vi "loopStop.vi"(8 "error in (no error)":errorcluster, 11 "Pixelfly in":refnum<class "PixelflySA.lvclass">) -> (0 "error out":errorcluster, 3 "Pixelfly out":refnum<class "PixelflySA.lvclass">)   [LabVIEW 2009, in "PixelflySA.lvclass"]
uses:
  PixelflySA.lvclass
  PixelflySA.lvclass/PixelflySA.ctl
  Channels.lvlib
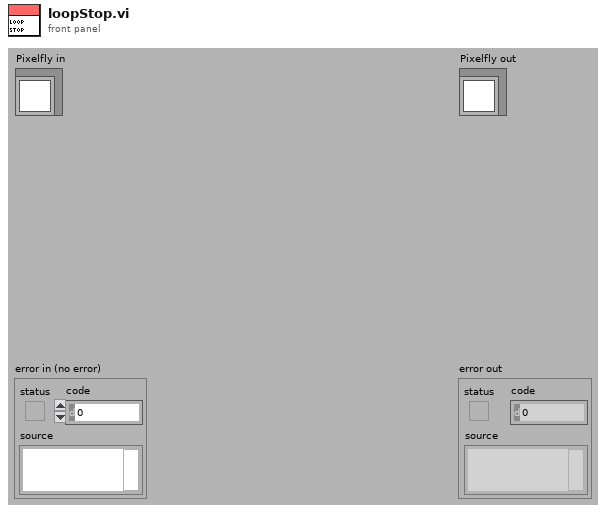
[diagram p1: front panel]
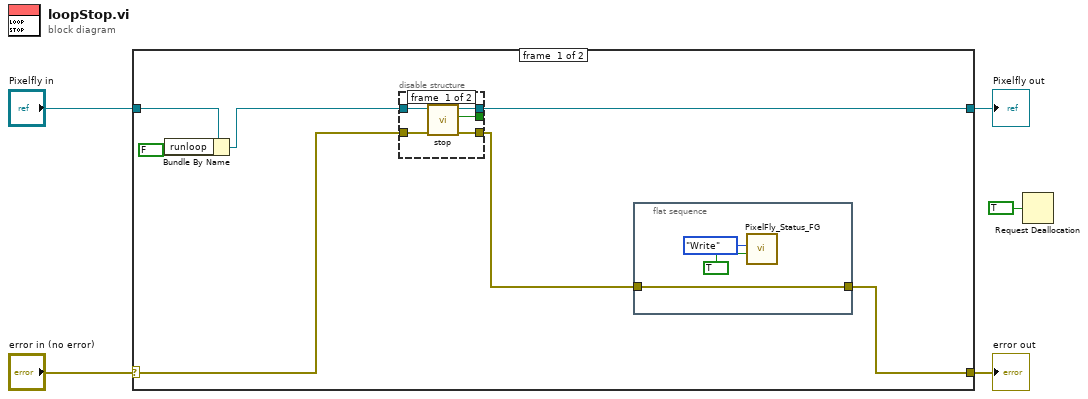
[diagram p0: block diagram]
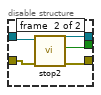
[diagram p2: hidden frame]
diagram:
  n1 = case shown="No Error" "error in (no error)" {
    selector: "error in (no error)" -> [w12 w27]
    tunnel: [w6 w27] -> w4
    tunnel: [w11 w26] -> w2
    tunnel: "Pixelfly in" -> [w9 w26]
    frame #0 {
      n2 = Bundle By Name(cluster=w9, "runloop"=FALSE) -> (w8:refnum<class "PixelflySA.lvclass">)
      n3 = disable-structure shown="Enabled" {
        disable-tunnel: w12 -> [w20 w23]
        disable-tunnel: [w19 w21] -> w7
        disable-tunnel: [w18 w22] -> _
        disable-tunnel: [w17 w25] -> w11
        disable-tunnel: w8 -> [w16 w24]
        frame #0 {
          n4 = call-dynamic "stop.vi"("error in (no error)"=w20, "Pixelfly in"=w16) -> ("error out"=w19:errorcluster, "stopped?"=w18:bool, "Pixelfly out"=w17:refnum<class "PixelflySA.lvclass">)  [unwired: 6 in, 1 out]
        }
        frame #1 {
          n5 = call-dynamic "stop2.vi"("error in (no error)"=w23, "Pixelfly in"=w24) -> ("error out"=w21:errorcluster, "stopped?"=w22:bool, "Pixelfly out"=w25:refnum<class "PixelflySA.lvclass">)  [unwired: 6 in, 1 out]
        }
      }
      n6 = flat-sequence {
        tunnel: w7 -> [w13]
        tunnel: [w13] -> w6
        frame #0 {
          n7 = call "PixelFly_Status_FG.vi"("stop"=TRUE, "Action"=enum16{"Write", "Read"}."Write") -> ()  [unwired: 9 in, 1 out]
        }
      }
    }
    frame #1 {
    }
  }
  "error out" <- w4
  "Pixelfly out" <- w2
  n8 = Request Deallocation(TRUE ("flag")) -> ()
